vi "Engine Out - Faults - Turbo Speed.vi"(11 "Turbo Speed [RPM]":sgl) -> ()   [LabVIEW 2015, in "ECS-RT.lvlib"]
uses:
  ECS-RT.lvlib
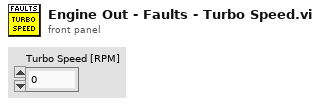
[diagram p1: front panel]
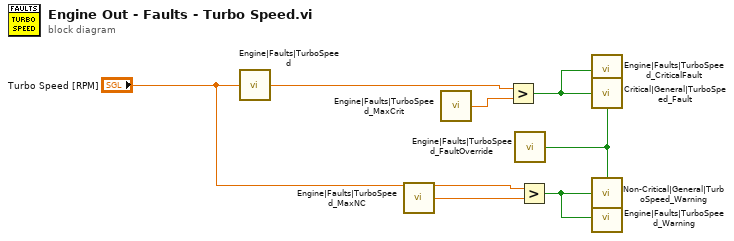
[diagram p0: block diagram]
diagram:
  n1 = call "Engine|Faults|TurboSpeed"("Value"="Turbo Speed [RPM]") -> ()
  n2 = call "Engine|Faults|TurboSpeed_MaxNC"() -> ("Value"=w5:sgl)
  n3 = call "Engine|Faults|TurboSpeed_MaxCrit"() -> ("Value"=w3:sgl)
  n4 = Greater?(x="Turbo Speed [RPM]", y=w3) -> (0:w4:bool)
  n5 = call "Engine|Faults|TurboSpeed_FaultOverride"() -> ("Value"=w1:bool)
  n6 = Greater?(x="Turbo Speed [RPM]", y=w5) -> (0:w6:bool)
  n7 = call "Engine|Faults|TurboSpeed_CriticalFault"("Value"=w4) -> ()
  n8 = call "Critical|General|TurboSpeed_Fault"("Fault"=w4, "Override (F)"=w1) -> ()  [unwired: 1 in]
  n9 = call "Non-Critical|General|TurboSpeed_Warning"("Fault"=w6, "Override (F)"=w1) -> ()  [unwired: 1 in]
  n10 = call "Engine|Faults|TurboSpeed_Warning"("Value"=w6) -> ()
